vi "Email Global.vi"(7 "Write (F)":bool, 11 "Send Email":bool) -> (3 "Send Email OUT":bool)   [LabVIEW 2013]
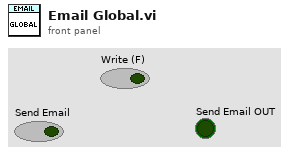
[diagram p1: front panel]
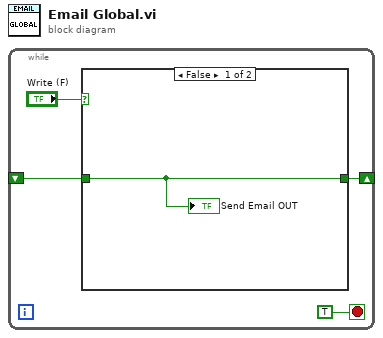
[diagram p0: block diagram]
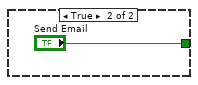
[diagram p2: hidden frame]
diagram:
  n1 = while {
    shift-right: [w2] -> _
    shift-left: _ -> [w1]
    stop <- TRUE stop-if-true
    n2 = case shown="False" "Write (F)" {
      tunnel: [w5 "Send Email"] -> w2
      tunnel: w1 -> [w5 _]
      frame False {
        "Send Email OUT" <- w5
      }
      frame True {
      }
    }
  }
